vi "Player Info.vi"(11 "Uno in":refnum<class "Uno.lvclass">) -> (0 "Defeat Speech":string, 1 "Victory Speech":string, 2 "Name":string, 3 "Uno out":refnum<class "Uno.lvclass">)   [LabVIEW 2015, in "Uno.lvclass"]
uses:
  Uno.lvclass
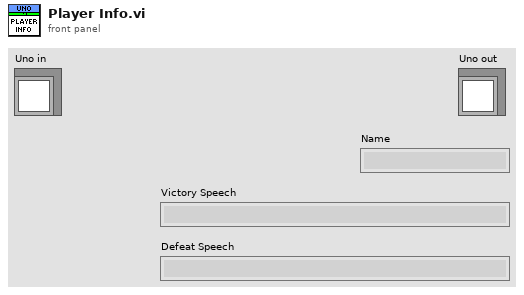
[diagram p1: front panel]
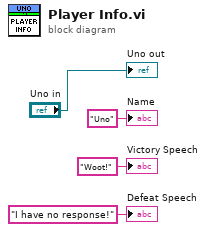
[diagram p0: block diagram]
diagram:
  "Uno out" <- "Uno in"
  "Name" <- "Uno" ("Name")
  "Victory Speech" <- "Woot!" ("Victory Speech")
  "Defeat Speech" <- "I have no response!" ("Defeat Speech")
